vi "BRig_dataLC_ENL_PreR_DelayOpt_l1.vi"() -> (2 "output_ENL_PreR_DelayOpt":i32)   [LabVIEW 2014]
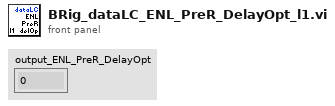
[diagram p1: front panel]
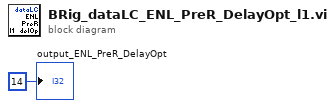
[diagram p0: block diagram]
diagram:
  "output_ENL_PreR_DelayOpt" <- 14 ("output_iBlock")
